vi "motorConfig.vi"(3 "Velocity":dbl=2.2 format="%#_6f", 4 "Acceleration":dbl=1.5, 5 "Device in":refnum<k24>) -> (2 "Device out":refnum<k24>)   [LabVIEW 2014]
doc: "André Romero - 2017\nandretec@ifsc.usp.br"
uses:
  C:/user-Lab/AndreTec/GITs/andretec/Thorlabs-Vector-Move/kinesisTec/Kinesis/Thorlabs.MotionControl.TCube.DCServoCLI.dll
  kinesisTec/Kinesis/Thorlabs.MotionControl.TCube.DCServoCLI.dll
  C:/user-Lab/AndreTec/GITs/andretec/Thorlabs-Vector-Move/kinesisTec/Kinesis/Thorlabs.MotionControl.GenericMotorCLI.dll
  kinesisTec/Kinesis/Thorlabs.MotionControl.GenericMotorCLI.dll
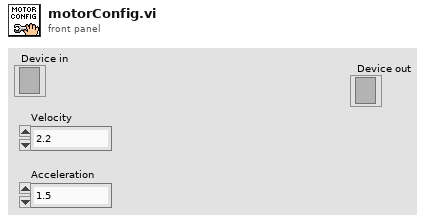
[diagram p1: front panel]
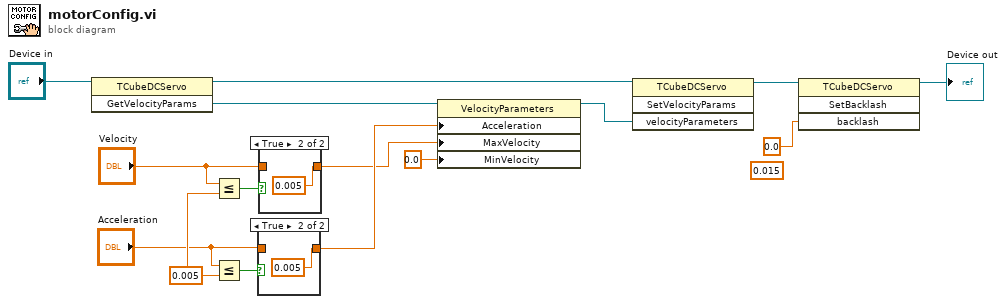
[diagram p0: block diagram]
diagram:
  w8 = 0.005 ("y")
  (unwired) 0.015 ("backlash")
  n1 = invoke class="TCubeDCServo" method="GetVelocityParams"(reference="Device in") -> (reference out=w14:refnum<k24>, "GetVelocityParams"=w9:refnum<k24>)  [unwired: 2 in, 1 out]
  n2 = Less Or Equal?(x="Velocity", y=w8) -> (x <= y?=w4:bool)
  n3 = Less Or Equal?(x="Acceleration", y=w8) -> (x <= y?=w7:bool)
  n4 = case shown="True" w7 {
    tunnel: "Acceleration" -> [w16 _]
    tunnel: [w16 0.005 ("y")] -> w5
    frame False {
    }
    frame True {
    }
  }
  n5 = case shown="True" w4 {
    tunnel: "Velocity" -> [w18 _]
    tunnel: [w18 0.005 ("y")] -> w3
    frame False {
    }
    frame True {
    }
  }
  n6 = property class="VelocityParameters"(reference=w9, "Acceleration"=w5, "MaxVelocity"=w3, "MinVelocity"=0.0) -> (reference out=w15:refnum<k24>)  [unwired: 1 in, 1 out]
  n7 = invoke class="TCubeDCServo" method="SetVelocityParams"(reference=w14, "velocityParameters"=w15) -> (reference out=w11:refnum<k24>)  [unwired: 2 in, 3 out]
  n8 = invoke class="TCubeDCServo" method="SetBacklash"(reference=w11, "backlash"=0.0) -> (reference out=→"Device out":refnum<k24>)  [unwired: 2 in, 3 out]
